vi "Deviated Result.vi"(0 "Device in":refnum<class "Device.lvclass">, 11 "Error in":errorcluster) -> (4 "Device out":refnum<class "Device.lvclass">, 15 "Error out":errorcluster)   [LabVIEW 2020, in "Device.lvclass"]
uses:
  Device.lvclass
  <vilib>/numeric/Random Number (Range) DBL.vi
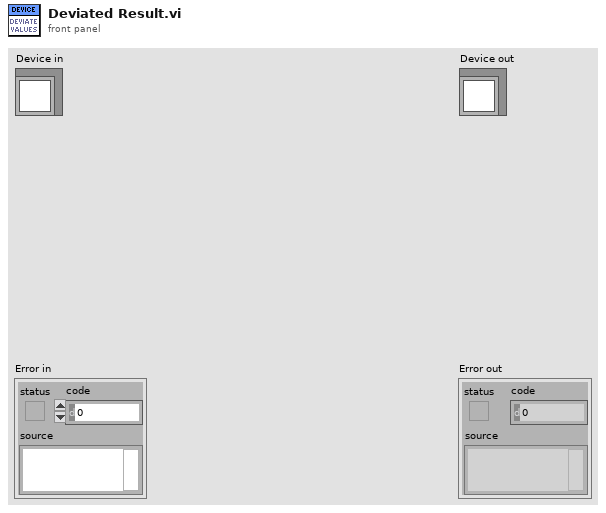
[diagram p1: front panel]
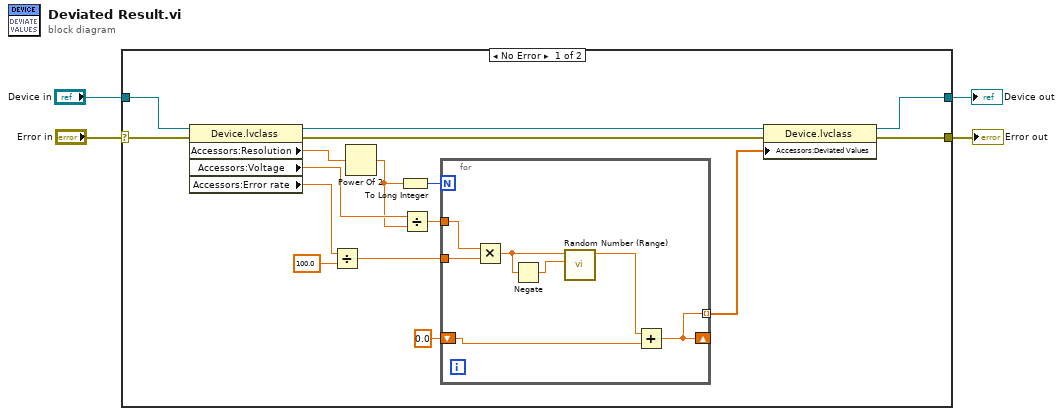
[diagram p0: block diagram]
diagram:
  n1 = case shown="No Error" "Error in" {
    selector: "Error in" -> [w20 w29]
    tunnel: [w8 w29] -> w3
    tunnel: [w5 w28] -> w1
    tunnel: "Device in" -> [w18 w28]
    frame No Error {
      n2 = property class="Device.lvclass"(reference=w18, error in=w20) -> (reference out=w7:refnum<class "Device.lvclass">, error out=w19:errorcluster, "Accessors:Resolution"=w17:dbl, "Accessors:Voltage"=w12:dbl, "Accessors:Error rate"=w16:dbl)
      n3 = Divide(x=w16, y=100.0) -> (x/y=w13:dbl)
      n4 = Power Of 2(x=w17) -> (2^x=w11:dbl)
      n5 = To Long Integer(number=w11) -> (32bit integer=w14:i32)
      n6 = Divide(x=w12, y=w11) -> (x/y=w10:dbl)
      n7 = for {
        N: w14 -> [_]
        tunnel: w13 -> [w26]
        tunnel: w10 -> [w27]
        shift-right: [w21] -> _
        shift-left: 0.0 -> [w22]
        tunnel: [w21] -> w6 mode=indexing
        n8 = Multiply(x=w27, y=w26) -> (x*y=w25:dbl)
        n9 = Negate(x=w25) -> (-x=w24:dbl)
        n10 = call-poly <vilib>:"Random Number (Range).vi"("lower bound (0)"=w24, "upper bound (100)"=w25) -> ("number"=w23:dbl)  [unwired: 9 in]
        n11 = Add(x=w23, y=w22) -> (x+y=w21:dbl)
      }
      n12 = property class="Device.lvclass"(reference=w7, error in=w19, "Accessors:Deviated Values"=w6) -> (reference out=w5:refnum<class "Device.lvclass">, error out=w8:errorcluster)
    }
    frame Error {
    }
  }
  "Error out" <- w3
  "Device out" <- w1
